vi "G#Debugger_GetObjectFromTag.vi"(0 "Objects dvr":refnum<data-value>, 1 "Tag":string, 2 "class attributes":bool, 5 "error in (no error)":errorcluster) -> (14 "Ref":refnum<class "G#Object.lvclass">, 15 "Found":bool, 19 "error out":errorcluster)   [LabVIEW 2017, in "G#Debugger.lvlib"]
uses:
  G#Debugger.lvlib
  G#Object/utils/G#Object_ClassInfoType.ctl
  G#Object/G#Object.lvclass
  G#Object/utils/G#Object_ObjectInfoType.ctl
  G#Object/utils/G#Object_CreateMethod.ctl
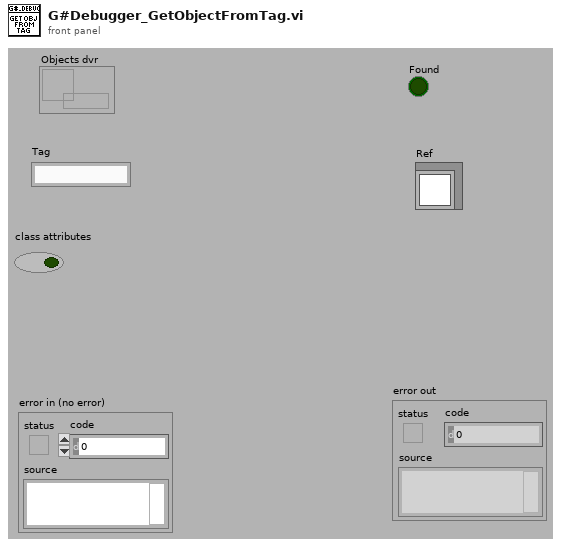
[diagram p1: front panel]
types:
  T1 = typedef "G#Object.lvclass/G#Object_ClassInfoType.ctl" = cluster{"ClassName":string, "ObjectInfo":T2[], "ObjectRefs":refnum<class "G#Object.lvclass">[], "TypeRef":refnum<class "G#Object.lvclass">}
  T2 = typedef "G#Object.lvclass/G#Object_ObjectInfoType.ctl" = cluster{"ObjectName":string, "ObjectID":u32, "Users":i32, "Counter":bool, "AttributeRefs":u32[], "FullClassName":string, "ClassName":string, "CreateMethod":T3, "GenericDestructorExists":bool, "Owner":string}
  T3 = typedef "G#Object.lvclass/G#Object_CreateMethod.ctl" = enum16{"Create", "Create or look up existing", "Look up existing"}
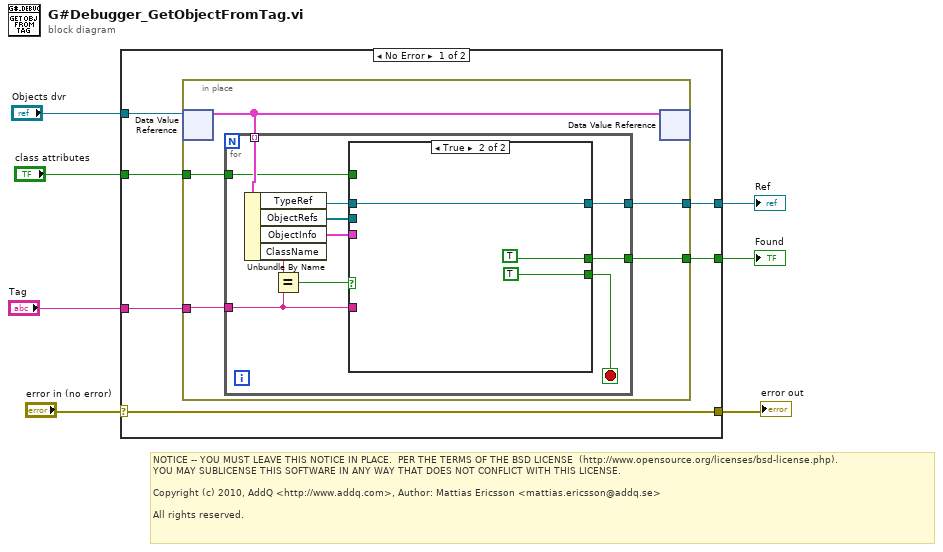
[diagram p0: block diagram]
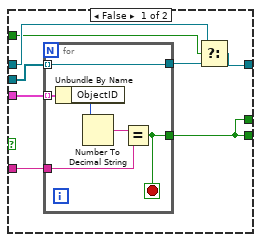
[diagram p2: hidden frame]
diagram:
  # "NOTICE -- YOU MUST LEAVE THIS NOTICE IN PLACE.  PER THE TERMS OF THE BSD LICENSE  (http://www.opensource.org/licenses/bsd-license.php).\nYOU MAY SUBLICENSE THIS SOFTWARE IN ANY WAY THAT DOES NOT CONFLICT WITH THIS LICENSE.\n\nCopyright (c) 2010, AddQ <http://www.addq.com>, Author: Mattias Ericsson <mattias.ericsson@addq.se>\n\nAll rights reserved."
  n1 = case shown="No Error" "error in (no error)" {
    selector: "error in (no error)" -> [w9 w47]
    tunnel: [w9 w47] -> w6
    tunnel: "Objects dvr" -> [w13 _]
    tunnel: "Tag" -> [w12 _]
    tunnel: [w11 _] -> w3
    tunnel: [w10 _] -> w2
    tunnel: "class attributes" -> [w8 _]
    frame No Error {
      n2 = in-place {
        in-place-border: w12 -> [w18]
        in-place-border: [w16] -> w11
        in-place-border: [w15] -> w10
        in-place-border: w8 -> [w14]
        n3 = in-place-dvr #1(w13) -> (w17:T1[])  [unwired: 1 out]
        n4 = for {
          tunnel: w17 -> [w29] mode=indexing
          tunnel: w18 -> [w26]
          tunnel: [w21] -> w16
          tunnel: [w24] -> w15
          tunnel: w14 -> [w19]
          stop <- w27 stop-if-true
          n5 = Unbundle By Name(w29) -> ("TypeRef"=w22:refnum<class "G#Object.lvclass">, "ObjectRefs"=w20:refnum<class "G#Object.lvclass">[], "ObjectInfo"=w28:T2[], "ClassName"=w25:string)
          n6 = Equal?(x=w25, y=w26) -> (x = y?=w23:bool)
          n7 = case shown="True" w23 {
            tunnel: w28 -> [w37 _]
            tunnel: [w35 TRUE] -> w27
            tunnel: w26 -> [w36 _]
            tunnel: [w32 w46] -> w24
            tunnel: w22 -> [w31 w46]
            tunnel: [w35 TRUE] -> w21
            tunnel: w20 -> [w34 _]
            tunnel: w19 -> [w30 _]
            frame False {
              n8 = for {
                tunnel: w37 -> [w43] mode=indexing
                tunnel: w36 -> [w40]
                tunnel: [w39] -> w35
                tunnel: [w38] -> w33
                tunnel: w34 -> [w38] mode=indexing
                stop <- w39 stop-if-true
                n9 = Unbundle By Name(w43) -> ("ObjectID"=w42:u32)
                n10 = Number To Decimal String(number=w42) -> (decimal integer string=w41:string)  [unwired: 1 in]
                n11 = Equal?(x=w41, y=w40) -> (x = y?=w39:bool)
              }
              n12 = Select(t=w31, s=w30, f=w33) -> (s? t:f=w32:refnum<class "G#Object.lvclass">)
            }
            frame True {
            }
          }
        }
        n13 = in-place-dvr #1(w17) -> ()  [unwired: 2 out]
      }
    }
    frame Error {
    }
  }
  "error out" <- w6
  "Found" <- w3
  "Ref" <- w2
